vi "P1_ADC_TEST_33600A_1122.vi"() -> ()   [LabVIEW 2015]
uses:
  E:/P1_ADC_TEST_2017/LabVIEW_1130/LBNE_DLL/LBNE_DLL/bin/Debug/LBNE_DLL.dll
  LBNE_Global .vi
  Agilent 3352X Series/Agilent 3352X Series.lvlib
panel:
  in  "y":bool
  in  "ext clk_choice":u8(slide)
  in  "default_right_clk2":T1={"RD/EN_OFF"=4.6e-07, "CLOCK"=5e-09, "ADC_OFF"=0.0, "ADC_WID"=6e-08, "MSB_OFF"=2e-07, "MSB_WID"=3e-07, "PERIOD"=5e-07, "LSB_FC_WID2"=5e-08, "LSB_FC_OFF1"=5e-08, "RD/EN_WID"=3e-08, "LSB_FC_WID1"=1.6e-07, "LSB_FC_OFF2"=4.5e-07, "LSB_S_WID"=5e-08, "LSB_S_OFF"=4.5e-07, "INV_RST"=TRUE, "INV_READ"=TRUE, "INV_MSB"=FALSE, "INV_LSB"=FALSE, "INV_LSB_1st"=FALSE, "Mult"=1.0} {"Mult" format="%#_6p"; "LSB_S_OFF" min=0.0 max=0.000655 step=1e-08 format="%#_6p"; "LSB_S_WID" min=1e-08 max=0.000655 step=1e-08 format="%#_6p"; "LSB_FC_OFF2" min=0.0 max=0.000655 step=1e-08 format="%#_6p"; "LSB_FC_WID1" min=1e-08 max=0.000655 step=1e-08 format="%#_6p"; "RD/EN_WID" min=1e-08 max=0.000655 step=1e-08 format="%#_6p"; "LSB_FC_OFF1" min=0.0 max=0.000655 step=1e-08 format="%#_6p"; "LSB_FC_WID2" min=1e-08 max=0.000655 step=1e-08 format="%#_6p"; "PERIOD" min=1e-08 max=0.000655 step=1e-08 format="%#_6p"; "MSB_WID" min=1e-08 max=0.000655 step=1e-08 format="%#_6p"; "MSB_OFF" min=0.0 max=0.000655 step=1e-08 format="%#_6p"; "ADC_WID" min=1e-08 max=0.000655 step=1e-08 format="%#_6p"; "ADC_OFF" min=0.0 max=0.000655 step=1e-08 format="%#_6p"; "CLOCK" format="%#_6p"; "RD/EN_OFF" min=0.0 max=0.000655 step=1e-08 format="%#_6p"}
  in  "default_left_clk1":T1={"RD/EN_OFF"=4.5e-07, "CLOCK"=5e-09, "ADC_OFF"=0.0, "ADC_WID"=4.99999999999996e-08, "MSB_OFF"=2e-07, "MSB_WID"=3e-07, "PERIOD"=5e-07, "LSB_FC_WID2"=5e-08, "LSB_FC_OFF1"=5e-08, "RD/EN_WID"=5e-08, "LSB_FC_WID1"=1.55e-07, "LSB_FC_OFF2"=4.5e-07, "LSB_S_WID"=5e-08, "LSB_S_OFF"=4.5e-07, "INV_RST"=TRUE, "INV_READ"=TRUE, "INV_MSB"=FALSE, "INV_LSB"=FALSE, "INV_LSB_1st"=FALSE, "Mult"=1.0} {"Mult" format="%#_6p"; "LSB_S_OFF" min=0.0 max=0.000655 step=1e-08 format="%#_6p"; "LSB_S_WID" min=1e-08 max=0.000655 step=1e-08 format="%#_6p"; "LSB_FC_OFF2" min=0.0 max=0.000655 step=1e-08 format="%#_6p"; "LSB_FC_WID1" min=1e-08 max=0.000655 step=1e-08 format="%#_6p"; "RD/EN_WID" min=1e-08 max=0.000655 step=1e-08 format="%#_6p"; "LSB_FC_OFF1" min=0.0 max=0.000655 step=1e-08 format="%#_6p"; "LSB_FC_WID2" min=1e-08 max=0.000655 step=1e-08 format="%#_6p"; "PERIOD" min=1e-08 max=0.000655 step=1e-08 format="%#_6p"; "MSB_WID" min=1e-08 max=0.000655 step=1e-08 format="%#_6p"; "MSB_OFF" min=0.0 max=0.000655 step=1e-08 format="%#_6p"; "ADC_WID" min=1e-08 max=0.000655 step=1e-08 format="%#_6p"; "ADC_OFF" min=0.0 max=0.000655 step=1e-08 format="%#_6p"; "CLOCK" format="%#_6p"; "RD/EN_OFF" min=0.0 max=0.000655 step=1e-08 format="%#_6p"}
  in  "Emerson_clk3":T1={"RD/EN_OFF"=4.8e-07, "CLOCK"=5e-09, "ADC_OFF"=0.0, "ADC_WID"=4.99999999999996e-08, "MSB_OFF"=2.3e-07, "MSB_WID"=2.7e-07, "PERIOD"=5e-07, "LSB_FC_WID2"=2e-08, "LSB_FC_OFF1"=5e-08, "RD/EN_WID"=2e-08, "LSB_FC_WID1"=1.9e-07, "LSB_FC_OFF2"=4.8e-07, "LSB_S_WID"=2e-08, "LSB_S_OFF"=4.8e-07, "INV_RST"=TRUE, "INV_READ"=TRUE, "INV_MSB"=FALSE, "INV_LSB"=FALSE, "INV_LSB_1st"=FALSE, "Mult"=1.0} {"Mult" format="%#_6p"; "LSB_S_OFF" min=0.0 max=0.000655 step=1e-08 format="%#_6p"; "LSB_S_WID" min=1e-08 max=0.000655 step=1e-08 format="%#_6p"; "LSB_FC_OFF2" min=0.0 max=0.000655 step=1e-08 format="%#_6p"; "LSB_FC_WID1" min=1e-08 max=0.000655 step=1e-08 format="%#_6p"; "RD/EN_WID" min=1e-08 max=0.000655 step=1e-08 format="%#_6p"; "LSB_FC_OFF1" min=0.0 max=0.000655 step=1e-08 format="%#_6p"; "LSB_FC_WID2" min=1e-08 max=0.000655 step=1e-08 format="%#_6p"; "PERIOD" min=1e-08 max=0.000655 step=1e-08 format="%#_6p"; "MSB_WID" min=1e-08 max=0.000655 step=1e-08 format="%#_6p"; "MSB_OFF" min=0.0 max=0.000655 step=1e-08 format="%#_6p"; "ADC_WID" min=1e-08 max=0.000655 step=1e-08 format="%#_6p"; "ADC_OFF" min=0.0 max=0.000655 step=1e-08 format="%#_6p"; "CLOCK" format="%#_6p"; "RD/EN_OFF" min=0.0 max=0.000655 step=1e-08 format="%#_6p"}
  in  "FILE PATH_IN":path=path "F:/P1_ADC_raw/P1_112616"
  in  "Set":bool
  in  "DC Offset (0 V)":dbl=0.5
  in  "Waveform":u16(ring)=5 items=["Sine"=0, "Square"=1, "Ramp"=2, "Noise"=3, "DC"=4, "Triangle"=5, "Pulse"=6, "Sinc"=11, "D-Lorentz"=12, "Gaussian"=13, "Expo Fall"=14, "Expo Rise"=15, "Haversine"=16]
  in  "Freq(Hz)":dbl=200.0
  in  "Amp (0.1 Vpp)":dbl=1.0
  out "path":path=path "F:/P1_ADC_raw/P1_111416/P1_4_01_0_0_clk3"
  out "concatenated string":string="F:\\P1_ADC_raw\\P1_111416\\P1_4_01_0_0_clk3/EXT_CLK_CFG.jpg"
  out "values to FPGA":T2={"33"=3, "32"=4, "31"=96, "30"=38, "29"=10, "28"=4, "27"=96, "26"=54, "25"=46, "24"=4, "23"=96, "22"=10, "21"=0, "20"=100}
  in  "EXT_set":T1={"RD/EN_OFF"=4.6e-07, "CLOCK"=5e-09, "ADC_OFF"=0.0, "ADC_WID"=6e-08, "MSB_OFF"=2e-07, "MSB_WID"=3e-07, "PERIOD"=5e-07, "LSB_FC_WID2"=5e-08, "LSB_FC_OFF1"=5e-08, "RD/EN_WID"=3e-08, "LSB_FC_WID1"=1.6e-07, "LSB_FC_OFF2"=4.5e-07, "LSB_S_WID"=5e-08, "LSB_S_OFF"=4.5e-07, "INV_RST"=TRUE, "INV_READ"=TRUE, "INV_MSB"=FALSE, "INV_LSB"=FALSE, "INV_LSB_1st"=FALSE, "Mult"=1.0} {"Mult" format="%#_6p"; "LSB_S_OFF" min=0.0 max=0.000655 step=1e-08 format="%#_6p"; "LSB_S_WID" min=1e-08 max=0.000655 step=1e-08 format="%#_6p"; "LSB_FC_OFF2" min=0.0 max=0.000655 step=1e-08 format="%#_6p"; "LSB_FC_WID1" min=1e-08 max=0.000655 step=1e-08 format="%#_6p"; "RD/EN_WID" min=1e-08 max=0.000655 step=1e-08 format="%#_6p"; "LSB_FC_OFF1" min=0.0 max=0.000655 step=1e-08 format="%#_6p"; "LSB_FC_WID2" min=1e-08 max=0.000655 step=1e-08 format="%#_6p"; "PERIOD" min=1e-08 max=0.000655 step=1e-08 format="%#_6p"; "MSB_WID" min=1e-08 max=0.000655 step=1e-08 format="%#_6p"; "MSB_OFF" min=0.0 max=0.000655 step=1e-08 format="%#_6p"; "ADC_WID" min=1e-08 max=0.000655 step=1e-08 format="%#_6p"; "ADC_OFF" min=0.0 max=0.000655 step=1e-08 format="%#_6p"; "CLOCK" format="%#_6p"; "RD/EN_OFF" min=0.0 max=0.000655 step=1e-08 format="%#_6p"}
  out "x+y":u8=1 format="%b"
  out "TP_RES":u32=39341825
  in  "FREQ":u16=600
  in  "DLY":u8=79
  in  "AMPL":u8=1 format="%x"
  out "Waveform Graph 4":u32[](graph)
  in  "stop":bool
  out "Newfile":bool=TRUE
  out "save_filename":string="F:\\P1_ADC_raw\\P1_111416\\P1_4_01_0_0_clk3\\P1_4_01_0_0_clk3_RT_2MHz_chnF_11_15_01_34.bin"
  out "filename_cfg":string="F:\\P1_ADC_raw\\P1_111416\\P1_4_01_0_0_clk3\\P1_4_01_0_0_clk3_RT_2MHz_chnF_11_15_01_34"
  in  "Sampling":bool
  in  "Temperature":bool=TRUE
  in  "SET CHN":T3={"D_offset"=0, "PDSR"=FALSE, "PCSR"=FALSE, "slp"=FALSE, "tst"=TRUE}
  out "Channel":string="F"
  out "Passed time":u32=19535
  out "start":u32=196967065
  out "UDP_CLEANUP":string="ok"
  in  "filename":string="P1_3_01_0_0" caption="file name"
  out "FILE PATH":path=path "F:/P1_ADC_raw/P1_111416/P1_4_01_0_0_clk3"
  out "Store_Data":bool=TRUE
  in  "lowlevel (V)":dbl=-0.05 format="%#_13g"
  in  "Frequency (1000 Hz)":dbl=0.05
  in  "Amplitude (1 Vpp)":dbl=1.8
  in  "VISA resource in":refnum<visa-resource-name>="USB0::0x0957::0x5707::MY53801762::INSTR"
  in  "Debug UDP enable":bool
  in  "Stop debug UDP":bool
  in  "ADDRESS":u16=19
  in  "DATA":u32=9 format="%x"
  in  "UDP WRITE":bool
  out "DATA 3":u32=9 format="%x"
  in  "ADDRESS 3":u16=19
  in  "UDP READ":bool
  out "ADC RB":u32[](array[numeric])=[3, 0, 0, 0, 0, 0, 0, 0, 4352, 3, 0, 0, 0, 0, 0, 0, 0, 4352, 3, 0, 0, 0, 0, 0, 0, 0, 4352, 3, 0, 0, 0, 0, 0, 0, 0, 4352] format="%x"
  out "ADC in":u32[](array[numeric])=[65537, 0, 0, 0, 0, 0, 0, 0, 2290124928, 65537, 0, 0, 0, 0, 0, 0, 0, 2290124928, 65537, 0, 0, 0, 0, 0, 0, 0, 2290124928, 65537, 0, 0, 0, 0, 0, 0, 0, 2290124928] format="%x"
  in  "CHANNEL":u8(slide)
  in  "SYNC":bool
  out "DATA SHIFT":u8[](array[numeric])=[6, 6, 6, 6, 6, 6, 6, 6] format="%x"
  out "ADC  CLK \nPHASE":bool[](array[boolean])=[TRUE, TRUE, TRUE, TRUE, TRUE, TRUE, TRUE, FALSE]
  in  "ADC_TM EN":bool
  in  "TEST EN":u32 format="%x"
  in  "TEST PAT":u32=279 format="%x"
  in  "samples 3":i32=1000
  in  "default samples":u32=10000
  in  "Remote Host":string="192.168.121.1"
  out "start_udp_IO":string="OK"
  out "LBNE_DLL_VERSION":u32=102
  in  "UDP/I2C":bool=TRUE
  out "ADC channel (indicator)":T4(array[cluster])=[{"D_offset"=0, "PDSR"=FALSE, "PCSR"=FALSE, "slp"=FALSE, "tst"=TRUE}, {"D_offset"=0, "PDSR"=FALSE, "PCSR"=FALSE, "slp"=FALSE, "tst"=FALSE}, {"D_offset"=0, "PDSR"=FALSE, "PCSR"=FALSE, "slp"=FALSE, "tst"=FALSE}, {"D_offset"=0, "PDSR"=FALSE, "PCSR"=FALSE, "slp"=FALSE, "tst"=FALSE}, {"D_offset"=0, "PDSR"=FALSE, "PCSR"=FALSE, "slp"=FALSE, "tst"=FALSE}, {"D_offset"=0, "PDSR"=FALSE, "PCSR"=FALSE, "slp"=FALSE, "tst"=FALSE}, {"D_offset"=0, "PDSR"=FALSE, "PCSR"=FALSE, "slp"=FALSE, "tst"=FALSE}, {"D_offset"=0, "PDSR"=FALSE, "PCSR"=FALSE, "slp"=FALSE, "tst"=FALSE}, {"D_offset"=0, "PDSR"=FALSE, "PCSR"=FALSE, "slp"=FALSE, "tst"=FALSE}, {"D_offset"=0, "PDSR"=FALSE, "PCSR"=FALSE, "slp"=FALSE, "tst"=FALSE}, {"D_offset"=0, "PDSR"=FALSE, "PCSR"=FALSE, "slp"=FALSE, "tst"=FALSE}, {"D_offset"=0, "PDSR"=FALSE, "PCSR"=FALSE, "slp"=FALSE, "tst"=FALSE}, {"D_offset"=0, "PDSR"=FALSE, "PCSR"=FALSE, "slp"=FALSE, "tst"=FALSE}, {"D_offset"=0, "PDSR"=FALSE, "PCSR"=FALSE, "slp"=FALSE, "tst"=FALSE}, {"D_offset"=0, "PDSR"=FALSE, "PCSR"=FALSE, "slp"=FALSE, "tst"=FALSE}, {"D_offset"=0, "PDSR"=FALSE, "PCSR"=FALSE, "slp"=FALSE, "tst"=FALSE}]
  in  "Global0":T5={"CLKG"=1, "FRQC"=0, "EN_GR"=0, "F0"=1, "F1"=0, "F2"=0, "F3"=0} {"F3" items=["0: IDL falling edge is delayed of 5-10ns after IDXM rising edge", "1: delay of 1 clock cycle on LVDS pin CLK"]; "F2" items=["0: the signal  generator on", "1: the signal  generator off"]; "F1" items=["0: a rising edge on LVDS pin ADC_CONV starts the sampling and readout", "1:the readout is compatible to V* version"]; "F0" items=["0: the ADC write clock is generated internally", "1: the ADC write clock is on LVDS pin IDXM"]; "FRQC" items=["0: 1 MHz", "1: 2 MHz "]; "CLKG" items=["0: ADC clocks from monostable", "1: External clocks", "2: ADC clocks from digital generator of FIFO", "3: ADC clocks from monostable"]; "EN_GR" items=["0: Disables offset current absorption", "1: Enables the offset current absorption"]}
  in  "Global1":T6={"F4"=1, "F5"=0, "sLSB"=0, "RES4-0(binary)"=0} {"RES4-0(binary)" items=["0", "1", "2", "3", "4", "5", "6", "7", "8", "9", "10", "11", "12", "13", "14", "15"]; "sLSB" items=["0: Full", "1: partial"]; "F5" items=["0: ADC data is selected and pipelined", "1: test data is selected and pipelined"]; "F4" items=["0: eanble F5", "1: CMOS pins CS and CLK controls the pipeline"]}
  out "ADC ARRAY":bool[](array[boolean])=[TRUE, FALSE, FALSE, FALSE, FALSE, FALSE, FALSE, FALSE, FALSE, FALSE, FALSE, FALSE, FALSE, FALSE, FALSE, FALSE, FALSE, FALSE, FALSE, FALSE, FALSE, FALSE, FALSE, FALSE, FALSE, FALSE, FALSE, FALSE, FALSE, FALSE, FALSE, FALSE, FALSE, FALSE, FALSE, FALSE, FALSE, FALSE, FALSE, FALSE, FALSE, FALSE, FALSE, FALSE, FALSE, FALSE, FALSE, FALSE, FALSE, FALSE, FALSE, FALSE, FALSE, FALSE, FALSE, FALSE, FALSE, FALSE, FALSE, FALSE, FALSE, FALSE, FALSE, FALSE, FALSE, FALSE, FALSE, FALSE, FALSE, FALSE, FALSE, FALSE, FALSE, FALSE, FALSE, FALSE, FALSE, FALSE, FALSE, FALSE, FALSE, FALSE, FALSE, FALSE, FALSE, FALSE, FALSE, FALSE, FALSE, FALSE, FALSE, FALSE, FALSE, FALSE, FALSE, FALSE, FALSE, FALSE, FALSE, FALSE, FALSE, FALSE, FALSE, FALSE, FALSE, FALSE, FALSE, FALSE, FALSE, FALSE, FALSE, FALSE, FALSE, FALSE, FALSE, FALSE, FALSE, FALSE, FALSE, FALSE, FALSE, FALSE, FALSE, FALSE, FALSE, FALSE, FALSE, FALSE, FALSE, FALSE, FALSE, FALSE, FALSE, FALSE, FALSE, TRUE, FALSE, FALSE, FALSE, TRUE, FALSE, FALSE, FALSE, TRUE, TRUE, FALSE, FALSE, FALSE, FALSE, FALSE, FALSE, FALSE, FALSE, FALSE, FALSE, FALSE, FALSE, FALSE, FALSE, FALSE, FALSE, FALSE, FALSE, FALSE, FALSE, FALSE, FALSE, FALSE, FALSE, FALSE, FALSE, FALSE, FALSE, FALSE, FALSE, FALSE, FALSE, FALSE, FALSE, FALSE, FALSE, FALSE, FALSE, FALSE, FALSE, FALSE, FALSE, FALSE, FALSE, FALSE, FALSE, FALSE, FALSE, FALSE, FALSE, FALSE, FALSE, FALSE, FALSE, FALSE, FALSE, FALSE, FALSE, FALSE, FALSE, FALSE, FALSE, FALSE, FALSE, FALSE, FALSE, FALSE, FALSE, FALSE, FALSE, FALSE, FALSE, FALSE, FALSE, FALSE, FALSE, FALSE, FALSE, FALSE, FALSE, FALSE, FALSE, FALSE, FALSE, FALSE, FALSE, FALSE, FALSE, FALSE, FALSE, FALSE, FALSE, FALSE, FALSE, FALSE, FALSE, FALSE, FALSE, FALSE, FALSE, FALSE, FALSE, FALSE, FALSE, FALSE, FALSE, FALSE, FALSE, FALSE, FALSE, FALSE, FALSE, FALSE, FALSE, FALSE, FALSE, FALSE, FALSE, FALSE, FALSE, FALSE, FALSE, FALSE, FALSE, FALSE, FALSE, FALSE, FALSE, FALSE, FALSE, FALSE, FALSE, FALSE, FALSE, TRUE, FALSE, FALSE, FALSE, TRUE, FALSE, FALSE, FALSE, TRUE, TRUE, FALSE, FALSE, FALSE, FALSE, FALSE, FALSE, FALSE, FALSE, FALSE, FALSE, FALSE, FALSE, FALSE, FALSE, FALSE, FALSE, FALSE, FALSE, FALSE, FALSE, FALSE, FALSE, FALSE, FALSE, FALSE, FALSE, FALSE, FALSE, FALSE, FALSE, FALSE, FALSE, FALSE, FALSE, FALSE, FALSE, FALSE, FALSE, FALSE, FALSE, FALSE, FALSE, FALSE, FALSE, FALSE, FALSE, FALSE, FALSE, FALSE, FALSE, FALSE, FALSE, FALSE, FALSE, FALSE, FALSE, FALSE, FALSE, FALSE, FALSE, FALSE, FALSE, FALSE, FALSE, FALSE, FALSE, FALSE, FALSE, FALSE, FALSE, FALSE, FALSE, FALSE, FALSE, FALSE, FALSE, FALSE, FALSE, FALSE, FALSE, FALSE, FALSE, FALSE, FALSE, FALSE, FALSE, FALSE, FALSE, FALSE, FALSE, FALSE, FALSE, FALSE, FALSE, FALSE, FALSE, FALSE, FALSE, FALSE, FALSE, FALSE, FALSE, FALSE, FALSE, FALSE, FALSE, FALSE, FALSE, FALSE, FALSE, FALSE, FALSE, FALSE, FALSE, FALSE, FALSE, FALSE, FALSE, FALSE, FALSE, FALSE, FALSE, FALSE, FALSE, FALSE, FALSE, FALSE, FALSE, FALSE, FALSE, FALSE, FALSE, FALSE, FALSE, TRUE, FALSE, FALSE, FALSE, TRUE, FALSE, FALSE, FALSE, TRUE, TRUE, FALSE, FALSE, FALSE, FALSE, FALSE, FALSE, FALSE, FALSE, FALSE, FALSE, FALSE, FALSE, FALSE, FALSE, FALSE, FALSE, FALSE, FALSE, FALSE, FALSE, FALSE, FALSE, FALSE, FALSE, FALSE, FALSE, FALSE, FALSE, FALSE, FALSE, FALSE, FALSE, FALSE, FALSE, FALSE, FALSE, FALSE, FALSE, FALSE, FALSE, FALSE, FALSE, FALSE, FALSE, FALSE, FALSE, FALSE, FALSE, FALSE, FALSE, FALSE, FALSE, FALSE, FALSE, FALSE, FALSE, FALSE, FALSE, FALSE, FALSE, FALSE, FALSE, FALSE, FALSE, FALSE, FALSE, FALSE, FALSE, FALSE, FALSE, FALSE, FALSE, FALSE, FALSE, FALSE, FALSE, FALSE, FALSE, FALSE, FALSE, FALSE, FALSE, FALSE, FALSE, FALSE, FALSE, FALSE, FALSE, FALSE, FALSE, FALSE, FALSE, FALSE, FALSE, FALSE, FALSE, FALSE, FALSE, FALSE, FALSE, FALSE, FALSE, FALSE, FALSE, FALSE, FALSE, FALSE, FALSE, FALSE, FALSE, FALSE, FALSE, FALSE, FALSE, FALSE, FALSE, FALSE, FALSE, FALSE, FALSE, FALSE, FALSE, FALSE, FALSE, FALSE, FALSE, FALSE, FALSE, FALSE, FALSE, FALSE, FALSE, FALSE, FALSE, TRUE, FALSE, FALSE, FALSE, TRUE, FALSE, FALSE, FALSE, TRUE, TRUE, FALSE, FALSE, FALSE, FALSE, FALSE, FALSE, FALSE, FALSE, FALSE, FALSE, FALSE, FALSE, FALSE, FALSE, FALSE, FALSE, FALSE, FALSE, FALSE, FALSE, FALSE, FALSE, FALSE, FALSE, FALSE, FALSE, FALSE, FALSE, FALSE, FALSE, FALSE, FALSE, FALSE, FALSE, FALSE, FALSE, FALSE, FALSE, FALSE, FALSE, FALSE, FALSE, FALSE, FALSE, FALSE, FALSE, FALSE, FALSE, FALSE, FALSE, FALSE, FALSE, FALSE, FALSE, FALSE, FALSE, FALSE, FALSE, FALSE, FALSE, FALSE, FALSE, FALSE, FALSE, FALSE, FALSE, FALSE, FALSE, FALSE, FALSE, FALSE, FALSE, FALSE, FALSE, FALSE, FALSE, FALSE, FALSE, FALSE, FALSE, FALSE, FALSE, FALSE, FALSE, FALSE, FALSE, FALSE, FALSE, FALSE, FALSE, FALSE, FALSE, FALSE, FALSE, FALSE, FALSE, FALSE, FALSE, FALSE, FALSE, FALSE, FALSE, FALSE, FALSE, FALSE, FALSE, FALSE, FALSE, FALSE, FALSE, FALSE, FALSE, FALSE, FALSE, FALSE, FALSE, FALSE, FALSE, FALSE, FALSE, FALSE, FALSE, FALSE, FALSE, FALSE, FALSE, FALSE, FALSE, FALSE, FALSE, FALSE, FALSE, FALSE, FALSE, TRUE, FALSE, FALSE, FALSE, TRUE, FALSE, FALSE, FALSE, TRUE, TRUE, FALSE, FALSE, FALSE, FALSE, FALSE, FALSE, FALSE, FALSE, FALSE, FALSE, FALSE, FALSE, FALSE, FALSE, FALSE, FALSE, FALSE, FALSE, FALSE, FALSE, FALSE, FALSE, FALSE, FALSE, FALSE, FALSE, FALSE, FALSE, FALSE, FALSE, FALSE, FALSE, FALSE, FALSE, FALSE, FALSE, FALSE, FALSE, FALSE, FALSE, FALSE, FALSE, FALSE, FALSE, FALSE, FALSE, FALSE, FALSE, FALSE, FALSE, FALSE, FALSE, FALSE, FALSE, FALSE, FALSE, FALSE, FALSE, FALSE, FALSE, FALSE, FALSE, FALSE, FALSE, FALSE, FALSE, FALSE, FALSE, FALSE, FALSE, FALSE, FALSE, FALSE, FALSE, FALSE, FALSE, FALSE, FALSE, FALSE, FALSE, FALSE, FALSE, FALSE, FALSE, FALSE, FALSE, FALSE, FALSE, FALSE, FALSE, FALSE, FALSE, FALSE, FALSE, FALSE, FALSE, FALSE, FALSE, FALSE, FALSE, FALSE, FALSE, FALSE, FALSE, FALSE, FALSE, FALSE, FALSE, FALSE, FALSE, FALSE, FALSE, FALSE, FALSE, FALSE, FALSE, FALSE, FALSE, FALSE, FALSE, FALSE, FALSE, FALSE, FALSE, FALSE, FALSE, FALSE, FALSE, FALSE, FALSE, FALSE, FALSE, FALSE, FALSE, TRUE, FALSE, FALSE, FALSE, TRUE, FALSE, FALSE, FALSE, TRUE, TRUE, FALSE, FALSE, FALSE, FALSE, FALSE, FALSE, FALSE, FALSE, FALSE, FALSE, FALSE, FALSE, FALSE, FALSE, FALSE, FALSE, FALSE, FALSE, FALSE, FALSE, FALSE, FALSE, FALSE, FALSE, FALSE, FALSE, FALSE, FALSE, FALSE, FALSE, FALSE, FALSE, FALSE, FALSE, FALSE, FALSE, FALSE, FALSE, FALSE, FALSE, FALSE, FALSE, FALSE, FALSE, FALSE, FALSE, FALSE, FALSE, FALSE, FALSE, FALSE, FALSE, FALSE, FALSE, FALSE, FALSE, FALSE, FALSE, FALSE, FALSE, FALSE, FALSE, FALSE, FALSE, FALSE, FALSE, FALSE, FALSE, FALSE, FALSE, FALSE, FALSE, FALSE, FALSE, FALSE, FALSE, FALSE, FALSE, FALSE, FALSE, FALSE, FALSE, FALSE, FALSE, FALSE, FALSE, FALSE, FALSE, FALSE, FALSE, FALSE, FALSE, FALSE, FALSE, FALSE, FALSE, FALSE, FALSE, FALSE, FALSE, FALSE, FALSE, FALSE, FALSE, FALSE, FALSE, FALSE, FALSE, FALSE, FALSE, FALSE, FALSE, FALSE, FALSE, FALSE, FALSE, FALSE, FALSE, FALSE, FALSE, FALSE, FALSE, FALSE, FALSE, FALSE, FALSE, FALSE, FALSE, FALSE, FALSE, FALSE, FALSE, FALSE, FALSE, TRUE, FALSE, FALSE, FALSE, TRUE, FALSE, FALSE, FALSE, TRUE, TRUE, FALSE, FALSE, FALSE, FALSE, FALSE, FALSE, FALSE, FALSE, FALSE, FALSE, FALSE, FALSE, FALSE, FALSE, FALSE, FALSE, FALSE, FALSE, FALSE, FALSE, FALSE, FALSE, FALSE, FALSE, FALSE, FALSE, FALSE, FALSE, FALSE, FALSE, FALSE, FALSE, FALSE, FALSE, FALSE, FALSE, FALSE, FALSE, FALSE, FALSE, FALSE, FALSE, FALSE, FALSE, FALSE, FALSE, FALSE, FALSE, FALSE, FALSE, FALSE, FALSE, FALSE, FALSE, FALSE, FALSE, FALSE, FALSE, FALSE, FALSE, FALSE, FALSE, FALSE, FALSE, FALSE, FALSE, FALSE, FALSE, FALSE, FALSE, FALSE, FALSE, FALSE, FALSE, FALSE, FALSE, FALSE, FALSE, FALSE, FALSE, FALSE, FALSE, FALSE, FALSE, FALSE, FALSE, FALSE, FALSE, FALSE, FALSE, FALSE, FALSE, FALSE, FALSE, FALSE, FALSE, FALSE, FALSE, FALSE, FALSE, FALSE, FALSE, FALSE, FALSE, FALSE, FALSE, FALSE, FALSE, FALSE, FALSE, FALSE, FALSE, FALSE, FALSE, FALSE, FALSE, FALSE, FALSE, FALSE, FALSE, FALSE, FALSE, FALSE, FALSE, FALSE, FALSE, FALSE, FALSE, FALSE, FALSE, FALSE, FALSE, FALSE, FALSE, TRUE, FALSE, FALSE, FALSE, TRUE, FALSE, FALSE, FALSE, TRUE]
  # "Generator setting"
  # "Default setting ( Don't change)"
  # "P1 ADC shift registers (144 bits)"
  # "1"
  # "2"
  # "3"
  # "4"
  # "5"
  # "6"
  # "7"
  # "8"
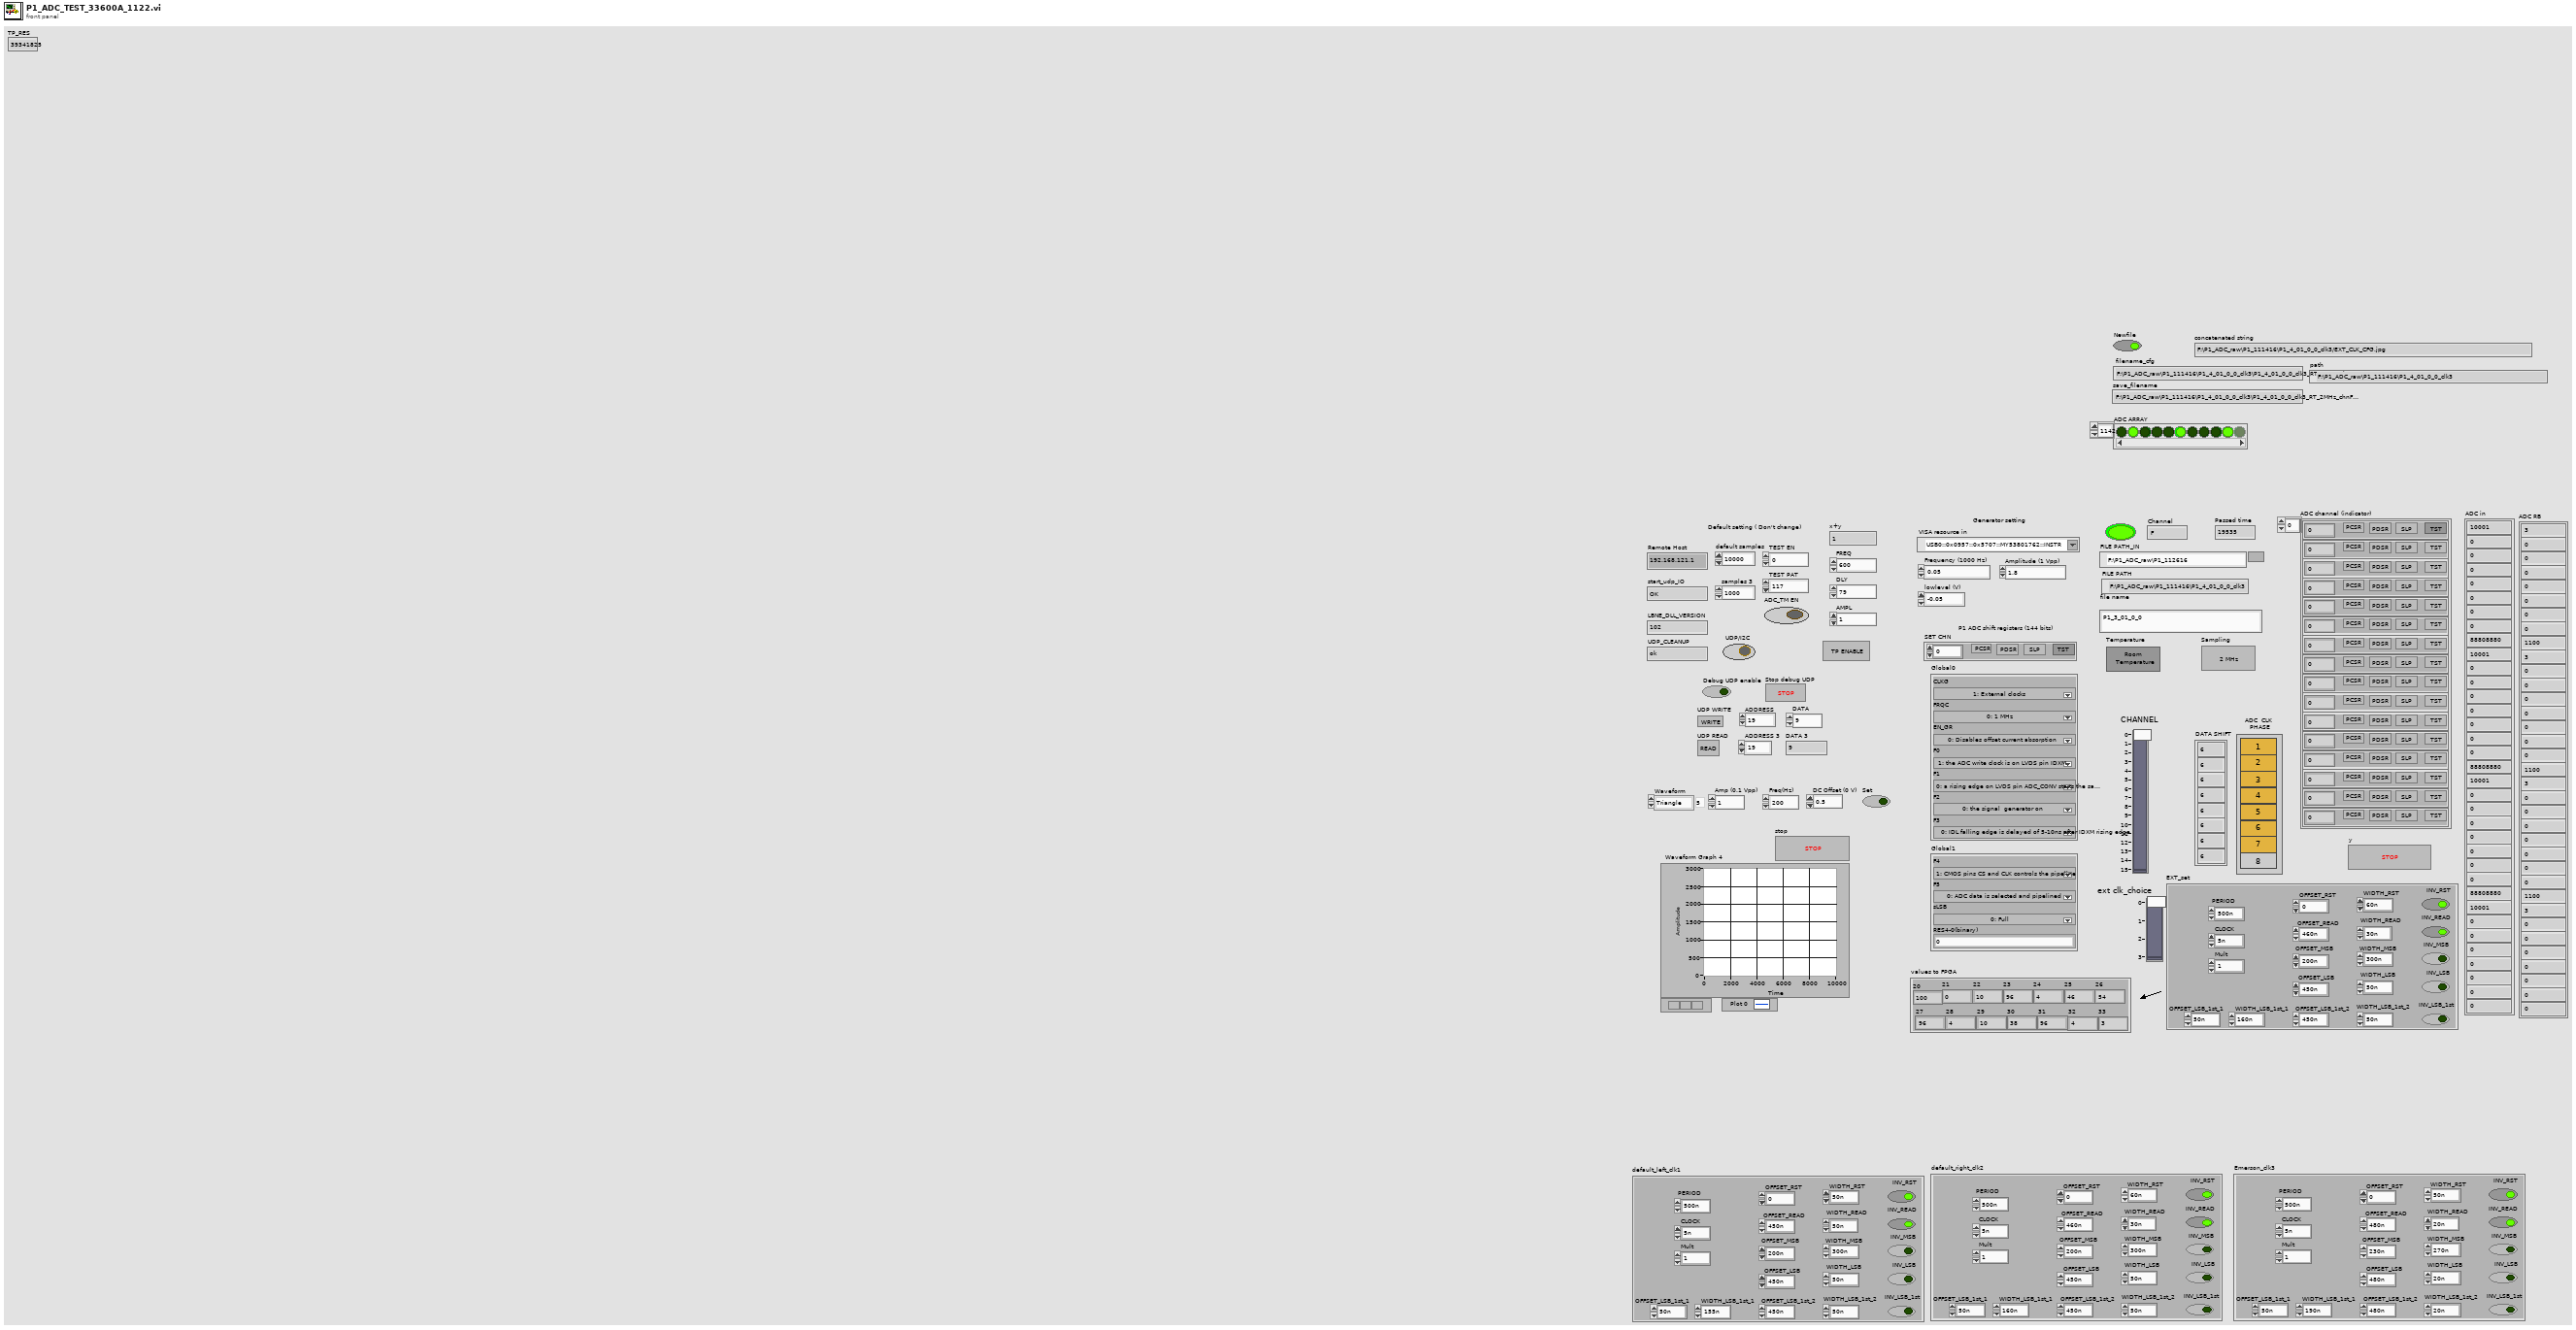
[diagram p1: front panel]
types:
  T1 = cluster{"RD/EN_OFF":dbl, "CLOCK":dbl, "ADC_OFF":dbl, "ADC_WID":dbl, "MSB_OFF":dbl, "MSB_WID":dbl, "PERIOD":dbl, "LSB_FC_WID2":dbl, "LSB_FC_OFF1":dbl, "RD/EN_WID":dbl, "LSB_FC_WID1":dbl, "LSB_FC_OFF2":dbl, "LSB_S_WID":dbl, "LSB_S_OFF":dbl, "INV_RST":bool, "INV_READ":bool, "INV_MSB":bool, "INV_LSB":bool, "INV_LSB_1st":bool, "Mult":dbl}
  T2 = cluster{"33":u16, "32":u16, "31":u16, "30":u16, "29":u16, "28":u16, "27":u16, "26":u16, "25":u16, "24":u16, "23":u16, "22":u16, "21":u16, "20":u16}
  T3 = cluster{"D_offset":u16, "PDSR":bool, "PCSR":bool, "slp":bool, "tst":bool}
  T4 = cluster{"D_offset":u16, "PDSR":bool, "PCSR":bool, "slp":bool, "tst":bool}[]
  T5 = cluster{"CLKG":u16, "FRQC":u16, "EN_GR":u16, "F0":u16, "F1":u16, "F2":u16, "F3":u16}
  T6 = cluster{"F4":u16, "F5":u16, "sLSB":u16, "RES4-0(binary)":u16}
  T7 = typedef "imagedata.ctl" = cluster{"image type":i32, "image depth":i32, "image":u8[], "mask":u8[], "colors":u32[], "Rectangle":cluster{"left":i16, "top":i16, "right":i16, "bottom":i16}}
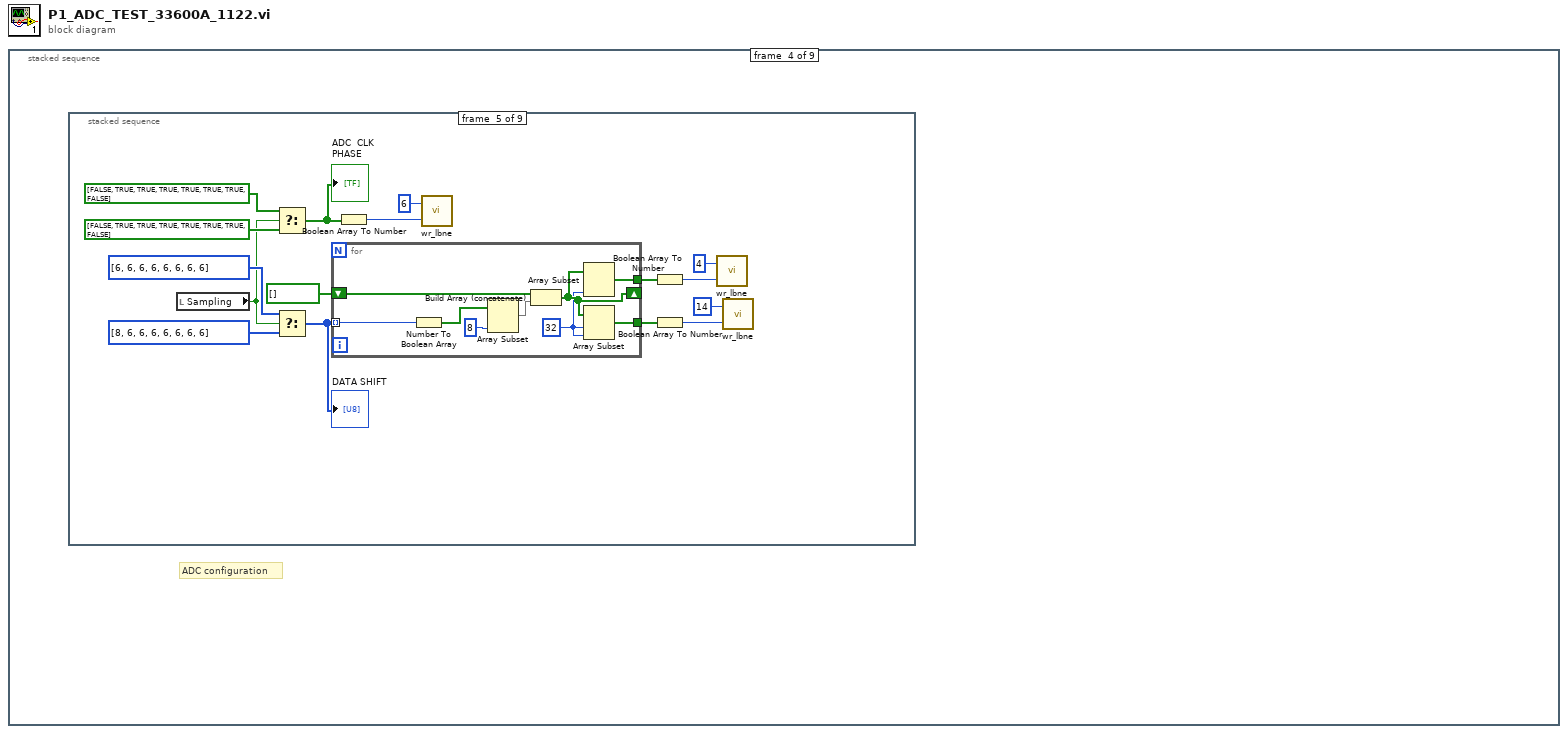
[diagram p0: block diagram]
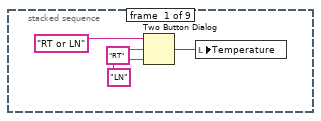
[diagram p2: hidden frame]
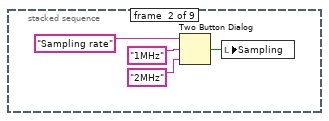
[diagram p3: hidden frame]
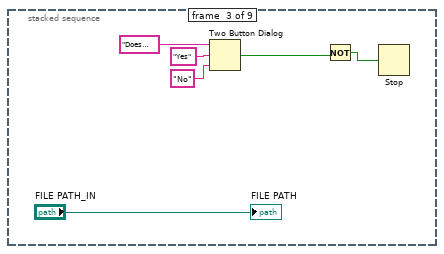
[diagram p4: hidden frame]
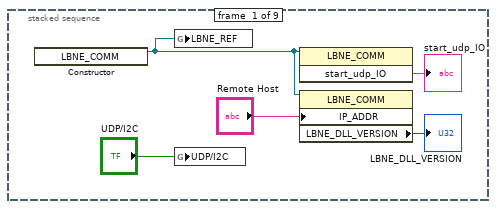
[diagram p5: hidden frame]
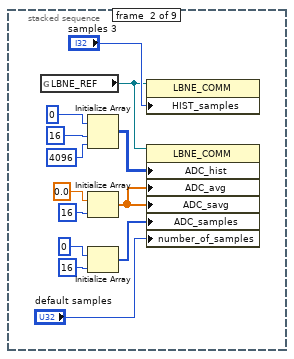
[diagram p6: hidden frame]
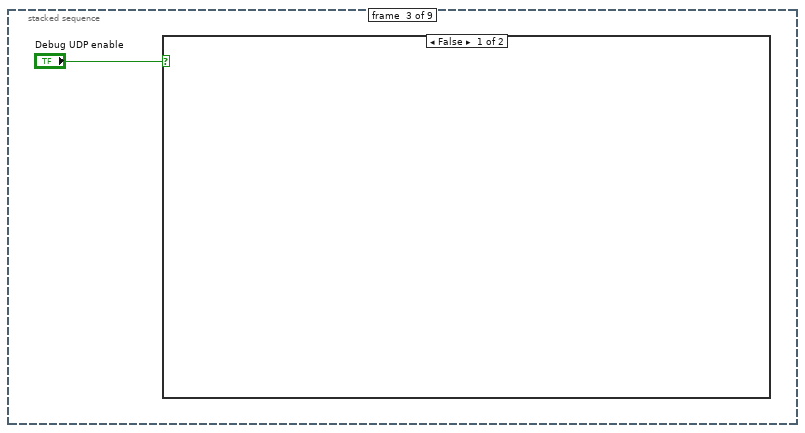
[diagram p7: hidden frame]
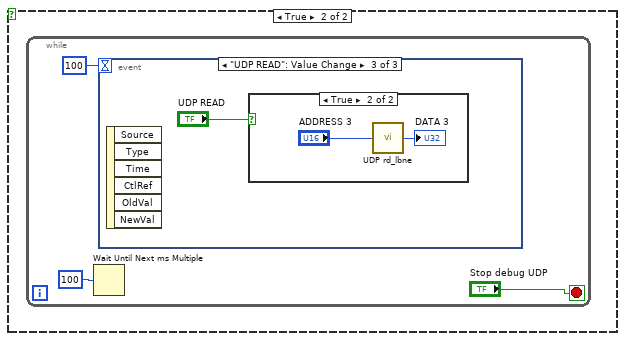
[diagram p8: hidden frame]
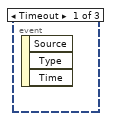
[diagram p9: hidden frame]
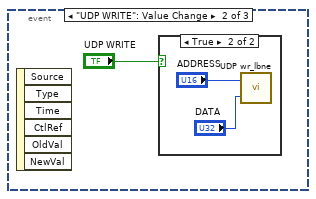
[diagram p10: hidden frame]
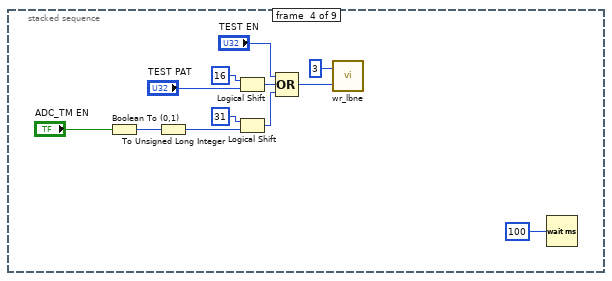
[diagram p13: hidden frame]
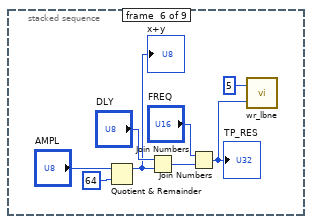
[diagram p14: hidden frame]
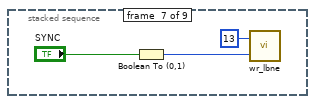
[diagram p15: hidden frame]
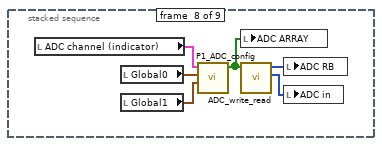
[diagram p16: hidden frame]
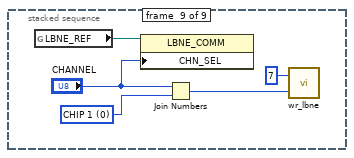
[diagram p17: hidden frame]
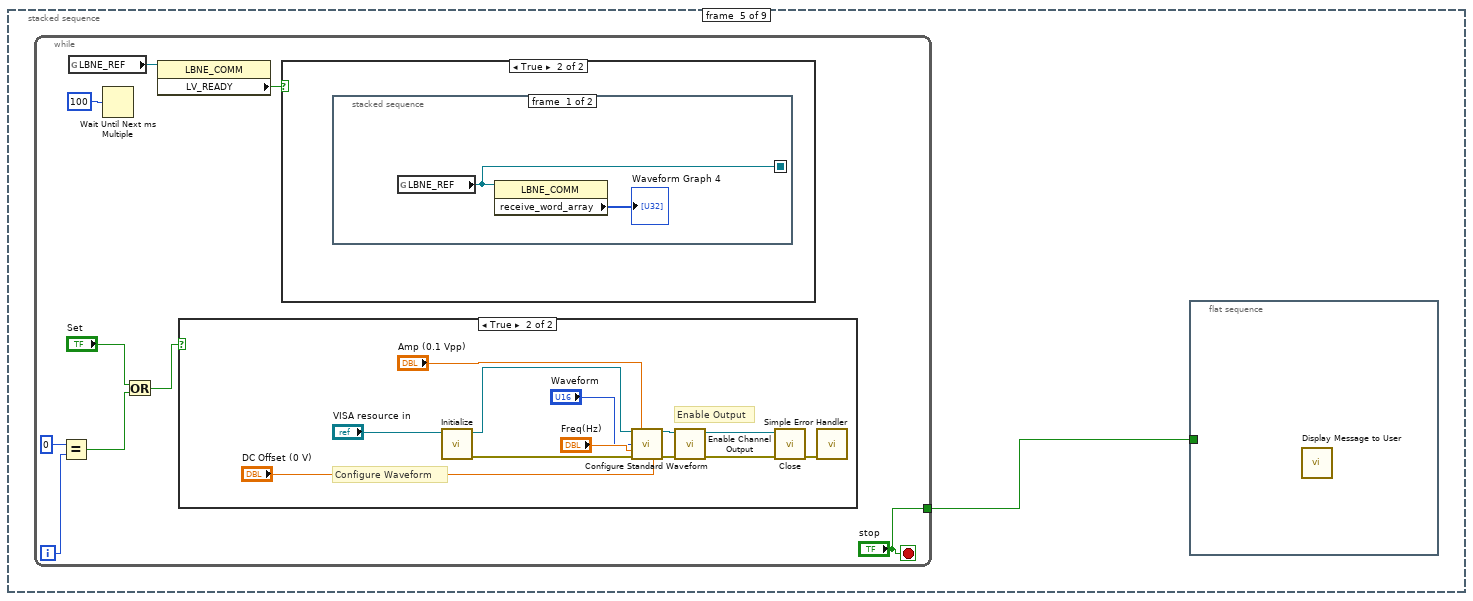
[diagram p18: hidden frame]
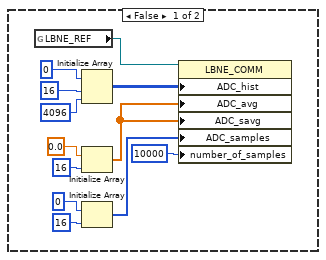
[diagram p20: hidden frame]
diagram:
  n1 = stacked-sequence {
    frame #0 {
      n2 = Two Button Dialog(message="RT or LN", 1:"LN" ("T button name (\"OK\")"), 2:"RT" ("F button name (\"Cancel\")")) -> (T button?=w4:bool)
      n3 = local write "Temperature"(w4) -> ()
    }
    frame #1 {
      n4 = Two Button Dialog(message="Sampling rate", 1:"2MHz" ("F button name (\"Cancel\")"), 2:"1MHz" ("T button name (\"OK\")")) -> (T button?=w5:bool)
      n5 = local write "Sampling"(w5) -> ()
    }
    frame #2 {
      n6 = Two Button Dialog(message="Does every setting is right?", 1:"No" ("F button name (\"Cancel\")"), 2:"Yes" ("T button name (\"OK\")")) -> (T button?=w13:bool)
      n7 = Not(x=w13) -> (.not. x?=w12:bool)
      n8 = Stop(stop? (T)=w12) -> ()
      "FILE PATH" <- "FILE PATH_IN"
    }
    frame #3 {
      # "ADC configuration"
      n9 = stacked-sequence {
        frame #0 {
          n10 = constructor class="LBNE_COMM"() -> (reference out=w15:refnum<k24>)  [unwired: 3 in, 2 out]
          n11 = global write "LBNE_Global .vi" "LBNE_REF"(w15) -> ()
          n12 = global write "LBNE_Global .vi" "UDP/I2C"("UDP/I2C") -> ()
          n13 = invoke class="LBNE_COMM" method="start_udp_IO"(reference=w15) -> ("start_udp_IO"=→"start_udp_IO":string)  [unwired: 2 in, 2 out]
          n14 = property class="LBNE_COMM"(reference=w15, "IP_ADDR"="Remote Host") -> ("LBNE_DLL_VERSION"=→"LBNE_DLL_VERSION":u32)  [unwired: 1 in, 2 out]
        }
        frame #1 {
          n15 = global read "LBNE_Global .vi" "LBNE_REF"() -> (w20:refnum<k24>)
          n16 = Initialize Array(u32 0 ("element"), 16 ("dimension size"), 4096 ("dimension size")) -> (w26:u32[][])
          n17 = Initialize Array(0.0 ("element"), 16 ("dimension size")) -> (w29:dbl[])
          n18 = Initialize Array(u32 0 ("element"), 16 ("dimension size")) -> (w31:u32[])
          n19 = property class="LBNE_COMM"(reference=w20, "HIST_samples"="samples 3") -> ()  [unwired: 1 in, 2 out]
          n20 = property class="LBNE_COMM"(reference=w20, "ADC_hist"=w26, "ADC_avg"=w29, "ADC_savg"=w29, "ADC_samples"=w31, "number_of_samples"="default samples") -> ()  [unwired: 1 in, 2 out]
        }
        frame #2 {
          n21 = case shown="False" "Debug UDP enable" {
            frame False {
            }
            frame True {
              n22 = while {
                stop <- "Stop debug UDP" stop-if-true
                n23 = Wait Until Next ms Multiple(millisecond multiple=u32 100) -> ()  [unwired: 1 out]
                n24 = event shown="[2] \"UDP READ\": Value Change" {
                  selector: _ -> [_ _ _]
                  dyn-events: _ -> [_ _ _]
                  timeout: 100 -> [_ _ _]
                  event Timeout {
                    n25 = event-data() -> ()  [unwired: 1 in, 3 out]
                  }
                  event "UDP WRITE": Value Change {
                    n26 = event-data() -> ()  [unwired: 1 in, 6 out]
                    n27 = case shown="True" "UDP WRITE" {
                      frame False {
                      }
                      frame True {
                        n28 = call "UDP wr_lbne.vi"("DATA"="DATA", "ADDRESS"="ADDRESS") -> ()  [unwired: 1 out]
                      }
                    }
                  }
                  event "UDP READ": Value Change {
                    n29 = event-data() -> ()  [unwired: 1 in, 6 out]
                    n30 = case shown="True" "UDP READ" {
                      frame False {
                      }
                      frame True {
                        n31 = call "UDP rd_lbne.vi"("ADDRESS 2"="ADDRESS 3") -> ("DATA 2"=→"DATA 3":u32)
                      }
                    }
                  }
                }
              }
            }
          }
        }
        frame #3 {
          n32 = Boolean To (0,1)(Boolean="ADC_TM EN") -> (0, 1=w53:i16)
          n33 = To Unsigned Long Integer(number=w53) -> (unsigned 32bit integer=w52:u32)
          n34 = Logical Shift(y=i16 16, x="TEST PAT") -> (x << y=w46:u32)
          n35 = Logical Shift(y=i16 31, x=w52) -> (x << y=w50:u32)
          n36 = Compound Arithmetic op=OR("TEST EN", w46, w50) -> (w54:u32)
          n37 = call "wr_lbne.vi"("DATA"=w54, "ADDRESS"=u16 3 ("address")) -> ()  [unwired: 1 out]
          n38 = Wait (ms)(milliseconds to wait=u32 100) -> ()  [unwired: 1 out]
        }
        frame #4 {
          n39 = local read "Sampling"() -> (w63:bool)
          n40 = Select(t=bool[] [FALSE, TRUE, TRUE, TRUE, TRUE, TRUE, TRUE, FALSE] ("ADC  CLK \nPHASE 2"), s=w63, f=bool[] [FALSE, TRUE, TRUE, TRUE, TRUE, TRUE, TRUE, FALSE] ("ADC  CLK \nPHASE 2")) -> (s? t:f=w66:bool[])
          "ADC  CLK \nPHASE" <- w66
          n41 = Select(t=u8[] [6, 6, 6, 6, 6, 6, 6, 6] ("DATA SHIFT 2"), s=w63, f=u8[] [8, 6, 6, 6, 6, 6, 6, 6] ("DATA SHIFT 2")) -> (s? t:f=w55:u8[])
          "DATA SHIFT" <- w55
          n42 = for {
            tunnel: w55 -> [w78] mode=indexing
            shift-right: [w73] -> _
            shift-left: bool[] [] -> [w75]
            tunnel: [w74] -> w59
            tunnel: [w71] -> w57
            w72 = 32 ("length")
            n43 = Number To Boolean Array(number=w78) -> (Boolean array=w77:bool[])
            n44 = Array Subset(array=w77, length=8) -> (w76:bool[])  [unwired: 1 in]
            n45 = Build Array (concatenate)(w75, w76) -> (w73:bool[])
            n46 = Array Subset(array=w73, length=w72) -> (w74:bool[])  [unwired: 1 in]
            n47 = Array Subset(array=w73, index=w72, length=w72) -> (w71:bool[])
          }
          n48 = Boolean Array To Number(Boolean array=w66) -> (number=w69:u32)
          n49 = call "wr_lbne.vi"("DATA"=w69, "ADDRESS"=u16 6 ("address")) -> ()  [unwired: 1 out]
          n50 = Boolean Array To Number(Boolean array=w59) -> (number=w60:u32)
          n51 = Boolean Array To Number(Boolean array=w57) -> (number=w56:u32)
          n52 = call "wr_lbne.vi"("DATA"=w60, "ADDRESS"=u16 4 ("address")) -> ()  [unwired: 1 out]
          n53 = call "wr_lbne.vi"("DATA"=w56, "ADDRESS"=u16 14 ("address")) -> ()  [unwired: 1 out]
        }
        frame #5 {
          n54 = Quotient & Remainder(x="AMPL", y=u8 64) -> (x-y*floor(x/y)=w80:u8)  [unwired: 1 out]
          "x+y" <- w80
          n55 = Join Numbers(hi="DLY", lo=w80) -> ((hi.lo)=w85:u16)
          n56 = Join Numbers(hi="FREQ", lo=w85) -> ((hi.lo)=w83:u32)
          "TP_RES" <- w83
          n57 = call "wr_lbne.vi"("DATA"=w83, "ADDRESS"=u16 5) -> ()  [unwired: 1 out]
        }
        frame #6 {
          n58 = Boolean To (0,1)(Boolean="SYNC") -> (0, 1=w89:i16)
          n59 = call "wr_lbne.vi"("DATA"=w89, "ADDRESS"=u16 13) -> ()  [unwired: 1 out]
        }
        frame #7 {
          n60 = local read "ADC channel (indicator)"() -> (w96:T4)
          n61 = local read "Global0"() -> (w95:T5)
          n62 = local read "Global1"() -> (w94:T6)
          n63 = call "P1_ADC_config.vi"("Global1"=w94, "Global0"=w95, "ADC channel"=w96) -> ("ADC ARRAY"=w91:bool[])  [unwired: 8 in]
          n64 = local write "ADC ARRAY"(w91) -> ()
          n65 = call "ADC_write_read.vi"("ADC  in"=w91) -> ("ADC in"=w92:u32[], "ADC out"=w93:u32[])  [unwired: 8 in, 1 out]
          n66 = local write "ADC RB"(w93) -> ()
          n67 = local write "ADC in"(w92) -> ()
        }
        frame #8 {
          w99 = u8 0 items=["CHIP 1", "CHIP 2", "CHIP 3", "CHIP 4", "CHIP 5", "CHIP 6", "CHIP 7", "CHIP 8"] ("CHIP")
          n68 = global read "LBNE_Global .vi" "LBNE_REF"() -> (w97:refnum<k24>)
          n69 = property class="LBNE_COMM"(reference=w97, "CHN_SEL"="CHANNEL") -> ()  [unwired: 1 in, 2 out]
          n70 = Join Numbers(hi="CHANNEL", lo=w99) -> ((hi.lo)=w100:u16)
          n71 = call "wr_lbne.vi"("DATA"=w100, "ADDRESS"=u16 7 ("address")) -> ()  [unwired: 1 out]
        }
      }
    }
    frame #4 {
      n72 = while {
        tunnel: ["stop"] -> w102
        i -> [w108]
        stop <- "stop" stop-if-true
        n73 = Equal?(x=0, y=w108) -> (x = y?=w106:bool)
        n74 = global read "LBNE_Global .vi" "LBNE_REF"() -> (w111:refnum<k24>)
        n75 = Wait Until Next ms Multiple(millisecond multiple=u32 100) -> ()  [unwired: 1 out]
        n76 = Or(x="Set", y=w106) -> (x .or. y?=w104:bool)
        n77 = property class="LBNE_COMM"(reference=w111) -> ("LV_READY"=w109:bool)  [unwired: 1 in, 2 out]
        n78 = case shown="True" w104 {
          frame False {
          }
          frame True {
            # "Enable Output"
            # "Configure Waveform"
            n79 = call "Initialize.vi"("VISA resource name"="VISA resource in") -> ("error out"=w118:errorcluster, "VISA resource name out"=w117:refnum<visa-resource-name>)  [unwired: 4 in, 5 out]
            n80 = call "Configure Standard Waveform.vi"("VISA resource name"=w117, "Amplitude (0.1 Vpp)"="Amp (0.1 Vpp)", "Waveform Function (0: Sine)"="Waveform", "Frequency/Sample Rate/Bandwidth (1000 Hz)"="Freq(Hz)", "error in (no error)"=w118, "DC Offset (0 V)"="DC Offset (0 V)") -> ("VISA resource name out"=w120:refnum<visa-resource-name>, "error out"=w119:errorcluster)  [unwired: 4 in, 4 out]
            n81 = call "Enable Channel Output.vi"("error in (no error)"=w119, "VISA resource name"=w120) -> ("error out"=w121:errorcluster, "VISA resource name out"=w122:refnum<visa-resource-name>)  [unwired: 3 in, 5 out]
            n82 = call "Close.vi"("error in (no error)"=w121, "VISA resource name"=w122) -> ("error out"=w123:errorcluster)  [unwired: 9 out]
            n83 = call <vilib>:"Simple Error Handler.vi"("error in (no error)"=w123) -> ()  [unwired: 1 in, 8 out]
          }
        }
        n84 = case shown="True" w109 {
          frame False {
            n85 = global read "LBNE_Global .vi" "LBNE_REF"() -> (w125:refnum<k24>)
            n86 = Initialize Array(u32 0 ("element"), 16 ("dimension size"), 4096 ("dimension size")) -> (w129:u32[][])
            n87 = Initialize Array(0.0 ("element"), 16 ("dimension size")) -> (w132:dbl[])
            n88 = Initialize Array(u32 0 ("element"), 16 ("dimension size")) -> (w134:u32[])
            n89 = property class="LBNE_COMM"(reference=w125, "ADC_hist"=w129, "ADC_avg"=w132, "ADC_savg"=w132, "ADC_samples"=w134, "number_of_samples"=u32 10000) -> ()  [unwired: 1 in, 2 out]
          }
          frame True {
            n90 = stacked-sequence {
              seq-local: [w136 _] -> [_ w139]
              frame #0 {
                n91 = global read "LBNE_Global .vi" "LBNE_REF"() -> (w136:refnum<k24>)
                n92 = property class="LBNE_COMM"(reference=w136) -> ("receive_word_array"=→"Waveform Graph 4":u32[])  [unwired: 1 in, 2 out]
              }
              frame #1 {
                n93 = property class="LBNE_COMM"(reference=w139, "LV_READY"=FALSE) -> ()  [unwired: 1 in, 2 out]
              }
            }
          }
        }
      }
      n94 = flat-sequence {
        tunnel: w102 -> [_]
        frame #0 {
          n95 = call "Display Message to User"() -> ()  [unwired: 10 in, 2 out]
        }
      }
    }
    frame #5 {
      n96 = local read "FILE PATH"() -> (w142:path)
      n97 = local read "filename"() -> (w143:string)
      n98 = Path To String(path=w142) -> (string=w149:string)
      n99 = Concatenate Strings(w149, "\\" ("string"), w143) -> (w148:string)
      n100 = String To Path(string=w148) -> (path=w146:path)
      n101 = call <vilib>:"Check if File or Folder Exists.vi"("path"=w146) -> ("file or folder exists?"=w145:bool, "dup path"=w144:path)  [unwired: 8 in, 1 out]
      n102 = Current VI's Path() -> (path=w153:path)
      n103 = case shown="False" w145 {
        tunnel: w144 -> [w160 w161]
        tunnel: [w159 w161] -> w140
        frame False {
          n104 = Create Folder(path (use dialog)=w160) -> (created path=w159:path)  [unwired: 2 in, 2 out]
        }
        frame True {
        }
      }
      n105 = Open VI Reference(vi path=w153) -> (vi reference=w154:refnum<vi>, error out=w155:errorcluster)  [unwired: 5 in]
      n106 = Path To String(path=w140) -> (string=w141:string)
      n107 = local write "FILE PATH"(w140) -> ()
      n108 = Concatenate Strings(w141, "/EXT_CLK_CFG.jpg" ("string")) -> (w151:string)
      "concatenated string" <- w151
      n109 = invoke on="Invoke Node" class="VI" method="FP.Get Image"(reference=w154, error in=w155) -> (reference out=w158:refnum<vi>, "image data"=w156:T7)  [unwired: 4 in, 4 out]
      n110 = String To Path(string=w151) -> (path=w152:path)
      n111 = call <vilib>:"Write JPEG File.vi"("image data"=w156, "path to JPEG file"=w152) -> ("error out"=w157:errorcluster)  [unwired: 8 in, 1 out]
      n112 = Close Reference(reference=w158) -> ()  [unwired: 1 in, 1 out]
      n113 = call <vilib>:"Simple Error Handler.vi"("error in (no error)"=w157) -> ()  [unwired: 4 in, 5 out]
    }
    frame #6 {
      w172 = 1 items=["1"=1, "2"=2] ("Cycle Count (1)")
      w175 = 0 items=["Triggered", "Gated"] ("Burst Mode (0: Triggered)")
      w183 = 2 items=["Sine"=0, "Square"=1, "Ramp"=2, "Noise"=3, "DC"=4, "Triangle"=5, "Pulse"=6, "Sinc"=11, "D-Lorentz"=12, "Gaussian"=13, "Expo Fall"=14, "Expo Rise"=15, "Haversine"=16] ("Waveform Function (0: Sine)")
      w181 = 0 items=["Degree", "Radian", "Second"] ("Angle Unit (0: Degree)")
      w164 = 1 items=["1"=1, "2"=2] ("Channel (1: 1)")
      # "Geneartor setting"
      n114 = Divide(x="Amplitude (1 Vpp)", y=2.0) -> (x/y=w178:dbl)
      n115 = Add(x=w178, y="lowlevel (V)") -> (x+y=w176:dbl)
      n116 = local read "VISA resource in"() -> (w162:refnum<visa-resource-name>)
      n117 = call "Initialize.vi"("VISA resource name"=w162) -> ("error out"=w185:errorcluster, "VISA resource name out"=w186:refnum<visa-resource-name>)  [unwired: 9 in]
      n118 = call "Configure Standard Waveform.vi"("VISA resource name"=w186, "Amplitude (0.1 Vpp)"="Amplitude (1 Vpp)", "Phase Angle (0 Degree)"=0.0, "Channel (1: 1)"=w164, "Waveform Function (0: Sine)"=w183, "Frequency/Sample Rate/Bandwidth (1000 Hz)"="Frequency (1000 Hz)", "error in (no error)"=w185, "Angle Unit (0: Degree)"=w181, "DC Offset (0 V)"=w176) -> ("VISA resource name out"=w169:refnum<visa-resource-name>, "error out"=w167:errorcluster)  [unwired: 5 in]
      n119 = call "Configure Channel Output.vi"("VISA resource name"=w169, "Output Impedance (50 Ohm)"=50.0, "Channel (1: 1)"=w164, "error in (no error)"=w167, "Enable Output (T: Enable)"=TRUE) -> ("VISA resource name out"=w168:refnum<visa-resource-name>, "error out"=w166:errorcluster)  [unwired: 9 in]
      n120 = call "Configure Burst.vi"("VISA resource name"=w168, "Burst Phase Angle (0 Degree)"=181.0, "Channel (1: 1)"=w164, "Burst Mode (0: Triggered)"=w175, "error in (no error)"=w166, "Infinite Cycle (T: Enable)"=FALSE, "Cycle Count (1)"=w172, "Burst Internal Period (10 ms)"=100.0) -> ("error out"=w170:errorcluster)  [unwired: 6 in, 1 out]
      n121 = flat-sequence {
        tunnel: w170 -> [w187]
        frame #0 {
          n122 = call <vilib>:"Simple Error Handler.vi"("error in (no error)"=w187) -> ()  [unwired: 4 in, 5 out]
        }
      }
    }
    frame #7 {
      # "Data acquisition"
      n123 = for {
        N: 16 -> [_]
        i -> [w192]
        stop <- w191 stop-if-true
        n124 = stacked-sequence {
          seq-local: [_ _ w241 _ _ _ _] -> [_ _ _ _ w251 _ _]
          seq-local: [_ _ _ _ w251 _ _] -> [_ _ _ _ _ w265 _]
          tunnel: w192 -> [w197 _ _ _ _ _ _]
          tunnel: w192 -> [_ w203 _ _ _ _ _]
          tunnel: [_ _ _ _ _ w265 _] -> w190
          frame #0 {
            n125 = local read "FILE PATH"() -> (w193:path)
            n126 = call "SAVE_PATH.vi"("chn_in"=w197, "Sampling"="Sampling", "Temperature"="Temperature", "filename"="filename", "folder"=w193) -> ("path"=→"path":path, "Newfile"=→"Newfile":bool, "save_filename"=→"save_filename":string, "Channel"=→"Channel":string, "filename_for_cfg"=→"filename_cfg":string)  [unwired: 2 in]
          }
          frame #1 {
            n127 = stacked-sequence {
              tunnel: w203 -> [w211 _]
              tunnel: w203 -> [_ w234]
              frame #0 {
                n128 = local write "CHANNEL"(w211) -> ()
                n129 = case shown="3" "ext clk_choice" {
                  tunnel: ["default_left_clk1" "default_right_clk2" "Emerson_clk3" "EXT_set"] -> w204
                  frame 0, Default {
                  }
                  frame 1 {
                  }
                  frame 2 {
                  }
                  frame 3 {
                  }
                }
                n130 = Replace Array Subset(array=T4 [{"D_offset"=0, "PDSR"=FALSE, "PCSR"=FALSE, "slp"=FALSE, "tst"=FALSE}, {"D_offset"=0, "PDSR"=FALSE, "PCSR"=FALSE, "slp"=FALSE, "tst"=FALSE}, {"D_offset"=0, "PDSR"=FALSE, "PCSR"=FALSE, "slp"=FALSE, "tst"=FALSE}, {"D_offset"=0, "PDSR"=FALSE, "PCSR"=FALSE, "slp"=FALSE, "tst"=FALSE}, {"D_offset"=0, "PDSR"=FALSE, "PCSR"=FALSE, "slp"=FALSE, "tst"=FALSE}, {"D_offset"=0, "PDSR"=FALSE, "PCSR"=FALSE, "slp"=FALSE, "tst"=FALSE}, {"D_offset"=0, "PDSR"=FALSE, "PCSR"=FALSE, "slp"=FALSE, "tst"=FALSE}, {"D_offset"=0, "PDSR"=FALSE, "PCSR"=FALSE, "slp"=FALSE, "tst"=FALSE}, {"D_offset"=0, "PDSR"=FALSE, "PCSR"=FALSE, "slp"=FALSE, "tst"=FALSE}, {"D_offset"=0, "PDSR"=FALSE, "PCSR"=FALSE, "slp"=FALSE, "tst"=FALSE}, {"D_offset"=0, "PDSR"=FALSE, "PCSR"=FALSE, "slp"=FALSE, "tst"=FALSE}, {"D_offset"=0, "PDSR"=FALSE, "PCSR"=FALSE, "slp"=FALSE, "tst"=FALSE}, {"D_offset"=0, "PDSR"=FALSE, "PCSR"=FALSE, "slp"=FALSE, "tst"=FALSE}, {"D_offset"=0, "PDSR"=FALSE, "PCSR"=FALSE, "slp"=FALSE, "tst"=FALSE}, {"D_offset"=0, "PDSR"=FALSE, "PCSR"=FALSE, "slp"=FALSE, "tst"=FALSE}, {"D_offset"=0, "PDSR"=FALSE, "PCSR"=FALSE, "slp"=FALSE, "tst"=FALSE}] ("ADC channel (default)"), new element="SET CHN", index=w211) -> (w206:T4)
                n131 = local write "ADC channel (indicator)"(w206) -> ()
                n132 = Unbundle By Name("Global0") -> ("CLKG"=w209:u16)
                n133 = for {
                  N: 2 -> [_]
                  tunnel: w206 -> [w232]
                  tunnel: "Global0" -> [w231]
                  tunnel: "Global1" -> [w230]
                  tunnel: [w229] -> w217
                  tunnel: [w228] -> w214
                  tunnel: [w227] -> w213
                  n134 = call "P1_ADC_config.vi"("Global1"=w230, "Global0"=w231, "ADC channel"=w232) -> ("ADC ARRAY"=w229:bool[])  [unwired: 8 in]
                  n135 = call "ADC_write_read.vi"("ADC  in"=w229) -> ("ADC in"=w228:u32[], "ADC out"=w227:u32[])  [unwired: 8 in, 1 out]
                }
                "ADC ARRAY" <- w217
                "ADC in" <- w214
                "ADC RB" <- w213
                n136 = Equal?(x=w209, y=u16 1) -> (x = y?=w207:bool)
                n137 = local read "filename_cfg"() -> (w212:string)
                n138 = case shown="True" w207 {
                  tunnel: w204 -> [_ w220]
                  frame False {
                  }
                  frame True {
                    n139 = call "ext_clk_config.vi"("EXT_set"=w220, "EN_ext_clk"=TRUE) -> ("values to FPGA"=→"values to FPGA":T2)  [unwired: 9 in]
                    n140 = local write "EXT_set"(w220) -> ()
                  }
                }
                n141 = call "save_adc_reg_cfg.vi"("filename_cfg"=w212, 10:"ADC in"=w213, 11:"ADC in"=w214) -> ()  [unwired: 9 in]
              }
              frame #1 {
                w236 = u8 0 items=["CHIP 1", "CHIP 2", "CHIP 3", "CHIP 4", "CHIP 5", "CHIP 6", "CHIP 7", "CHIP 8"] ("CHIP")
                n142 = To Unsigned Byte Integer(number=w234) -> (unsigned 8bit integer=w235:u8)
                n143 = global read "LBNE_Global .vi" "LBNE_REF"() -> (w233:refnum<k24>)
                n144 = property class="LBNE_COMM"(reference=w233, "CHN_SEL"=w235) -> ()  [unwired: 1 in, 2 out]
                n145 = Join Numbers(hi=w235, lo=w236) -> ((hi.lo)=w237:u16)
                n146 = call "wr_lbne.vi"("DATA"=w237, "ADDRESS"=u16 7 ("address")) -> ()  [unwired: 1 out]
              }
            }
          }
          frame #2 {
            n147 = local read "save_filename"() -> (w240:string)
            n148 = local read "Newfile"() -> (w239:bool)
            n149 = case shown="True" w239 {
              tunnel: w240 -> [_ w243]
              frame False {
              }
              frame True {
                n150 = global read "LBNE_Global .vi" "LBNE_REF"() -> (w242:refnum<k24>)
                n151 = invoke class="LBNE_COMM" method="open_file"(reference=w242, "File_name"=w243) -> ()  [unwired: 2 in, 4 out]
              }
            }
            n152 = Not(x=w239) -> (.not. x?=w241:bool)
          }
          frame #3 {
            n153 = stacked-sequence {
              frame #0 {
                w247 = 3 items=["Immediate", "External", "Timer", "Bus"] ("Trigger Source (0: Immediate)")
                w248 = 1 items=["1"=1, "2"=2] ("Channel (1: 1)")
                n154 = local read "VISA resource in"() -> (w249:refnum<visa-resource-name>)
                n155 = call "Configure Trigger.vi"("Count Number (1)"=1, "Trigger Source (0: Immediate)"=w247, "Channel (1: 1)"=w248, "VISA resource name"=w249) -> ("error out"=w244:errorcluster, "VISA resource name out"=w245:refnum<visa-resource-name>)  [unwired: 6 in]
                n156 = call "Send Software Trigger.vi"("error in (no error)"=w244, "VISA resource name"=w245) -> ()  [unwired: 8 in, 2 out]
              }
              frame #1 {
                n157 = Tick Count (ms)() -> (millisecond timer value=→"start":u32)
              }
            }
          }
          frame #4 {
            n158 = case shown="False" w251 {
              frame False {
                n159 = while {
                  stop <- w258 stop-if-true
                  n160 = Wait Until Next ms Multiple(millisecond multiple=u32 50) -> ()  [unwired: 1 out]
                  n161 = global read "LBNE_Global .vi" "LBNE_REF"() -> (w257:refnum<k24>)
                  n162 = property class="LBNE_COMM"(reference=w257) -> ("Store_Data"=→"Store_Data":bool)  [unwired: 1 in, 2 out]
                  n163 = local read "Frequency (1000 Hz)"() -> (w260:dbl)
                  n164 = local read "start"() -> (w261:u32)
                  n165 = Tick Count (ms)() -> (millisecond timer value=w262:u32)
                  n166 = Subtract(x=w262, y=w261) -> (x-y=w256:u32)
                  "Passed time" <- w256
                  n167 = Divide(x=1000.0, y=w260) -> (x/y=w254:dbl)
                  n168 = Add(x=u32 2000 ("y"), y=w254) -> (x+y=w252:dbl)
                  n169 = To Unsigned Long Integer(number=w256) -> (unsigned 32bit integer=w255:u32)
                  n170 = Greater Or Equal?(x=w255, y=w252) -> (x >= y?=w258:bool)
                }
              }
              frame True {
              }
            }
          }
          frame #5 {
            n171 = case shown="False" w265 {
              frame False {
                n172 = global read "LBNE_Global .vi" "LBNE_REF"() -> (w266:refnum<k24>)
                n173 = invoke class="LBNE_COMM" method="open_file"(reference=w266, "File_name"="") -> ()  [unwired: 2 in, 4 out]
              }
              frame True {
              }
            }
          }
          frame #6 {
            n174 = Wait (ms)(milliseconds to wait=u32 1000 ("millisecond multiple")) -> ()  [unwired: 1 out]
          }
        }
        n175 = Or(x=w190, y="y") -> (x .or. y?=w191:bool)
      }
    }
    frame #8 {
      # "Stop"
      n176 = stacked-sequence {
        frame #0 {
          n177 = global read "LBNE_Global .vi" "LBNE_REF"() -> (w270:refnum<k24>)
          n178 = invoke class="LBNE_COMM" method="UDP_CLEANUP"(reference=w270) -> ("UDP_CLEANUP"=→"UDP_CLEANUP":string)  [unwired: 2 in, 2 out]
          n179 = local read "VISA resource in"() -> (w271:refnum<visa-resource-name>)
          n180 = call "Close.vi"("VISA resource name"=w271) -> ()  [unwired: 10 in, 1 out]
          "ADC channel (indicator)" <- T4 [{"D_offset"=0, "PDSR"=FALSE, "PCSR"=FALSE, "slp"=FALSE, "tst"=TRUE}, {"D_offset"=0, "PDSR"=FALSE, "PCSR"=FALSE, "slp"=FALSE, "tst"=FALSE}, {"D_offset"=0, "PDSR"=FALSE, "PCSR"=FALSE, "slp"=FALSE, "tst"=FALSE}, {"D_offset"=0, "PDSR"=FALSE, "PCSR"=FALSE, "slp"=FALSE, "tst"=FALSE}, {"D_offset"=0, "PDSR"=FALSE, "PCSR"=FALSE, "slp"=FALSE, "tst"=FALSE}, {"D_offset"=0, "PDSR"=FALSE, "PCSR"=FALSE, "slp"=FALSE, "tst"=FALSE}, {"D_offset"=0, "PDSR"=FALSE, "PCSR"=FALSE, "slp"=FALSE, "tst"=FALSE}, {"D_offset"=0, "PDSR"=FALSE, "PCSR"=FALSE, "slp"=FALSE, "tst"=FALSE}, {"D_offset"=0, "PDSR"=FALSE, "PCSR"=FALSE, "slp"=FALSE, "tst"=FALSE}, {"D_offset"=0, "PDSR"=FALSE, "PCSR"=FALSE, "slp"=FALSE, "tst"=FALSE}, {"D_offset"=0, "PDSR"=FALSE, "PCSR"=FALSE, "slp"=FALSE, "tst"=FALSE}, {"D_offset"=0, "PDSR"=FALSE, "PCSR"=FALSE, "slp"=FALSE, "tst"=FALSE}, {"D_offset"=0, "PDSR"=FALSE, "PCSR"=FALSE, "slp"=FALSE, "tst"=FALSE}, {"D_offset"=0, "PDSR"=FALSE, "PCSR"=FALSE, "slp"=FALSE, "tst"=FALSE}, {"D_offset"=0, "PDSR"=FALSE, "PCSR"=FALSE, "slp"=FALSE, "tst"=FALSE}, {"D_offset"=0, "PDSR"=FALSE, "PCSR"=FALSE, "slp"=FALSE, "tst"=FALSE}] ("ADC channel (indicator)")
        }
        frame #1 {
          w273 = u8 0 items=["CHN 0", "CHN 1", "CHN 2", "CHN 3", "CHN 4", "CHN 5", "CHN 6", "CHN 7", "CHN 8", "CHN 9", "CHN 10", "CHN 11", "CHN 12", "CHN 13", "CHN 14", "CHN 15"] ("CHANNEL")
          n181 = Wait Until Next ms Multiple(millisecond multiple=u32 1200) -> ()  [unwired: 1 out]
          n182 = local write "CHANNEL"(w273) -> ()
        }
      }
    }
  }
